vi "test Convert File Extension.vi"() -> ()   [LabVIEW 2017]
uses:
  049c2730-d305-4f14-8b30-2d1737075706.vi
  45676f0a-75d5-47ce-b3fc-46d64fd4f536.vi
  f7c2043c-194c-414b-9d0b-117c10e17b47.vi
panel:
  out "new filename 3":path
  out "new filename 2":path
  out "new filename":string
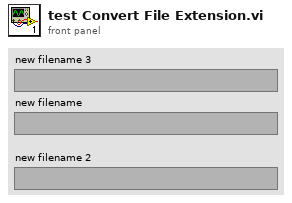
[diagram p1: front panel]
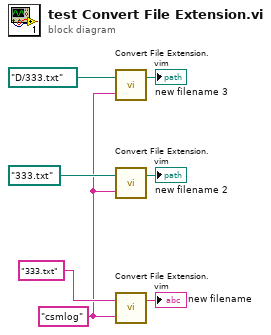
[diagram p0: block diagram]
diagram:
  w1 = "csmlog" ("new ending (none)")
  n1 = call "Convert File Extension.vim"("new ending (none)"=w1, "String/Path"=path "D:/333.txt") -> ("new filename"=→"new filename 3":path)  [unwired: 1 out]
  n2 = call "Convert File Extension.vim"("new ending (none)"=w1, "String/Path"=path "333.txt") -> ("new filename"=→"new filename 2":path)  [unwired: 1 out]
  n3 = call "Convert File Extension.vim"("new ending (none)"=w1, "String/Path"="333.txt") -> ("new filename"=→"new filename":string)  [unwired: 1 out]
